vi "LoadCallibrationResults.vi"() -> (1 "Peak coarse":dbl, 2 "Peak right":dbl, 3 "Peak left":dbl)   [LabVIEW 2013]
uses:
  <vilib>/Utility/file.llb/Read From Spreadsheet File (DBL).vi
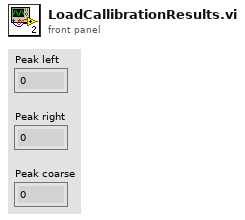
[diagram p1: front panel]
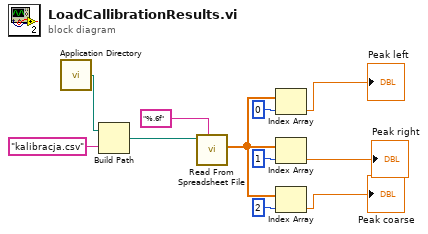
[diagram p0: block diagram]
diagram:
  n1 = call <vilib>:"Application Directory.vi"() -> ("Application Directory"=w1:path)
  n2 = Build Path(base path=w1, name or relative path="kalibracja.csv") -> (appended path=w3:path)
  n3 = call-poly <vilib>:"Read From Spreadsheet File.vi"("format (%.3f)"="%.6f", "file path (dialog if empty)"=w3) -> ("first row"=w6:dbl[])  [unwired: 5 in, 4 out]
  n4 = Index Array(array=w6, index=0) -> (element=→"Peak left":dbl)
  n5 = Index Array(array=w6, index=1) -> (element=→"Peak right":dbl)
  n6 = Index Array(array=w6, index=2) -> (element=→"Peak coarse":dbl)
